vi "Measurement FileGLobal FGV.vi"(0 "New Measurements":T1, 2 "Enum":T2(ring), 11 "Error In":errorcluster) -> (4 "Combined Measurements":T1, 15 "Error Out":errorcluster)   [LabVIEW 2013]
uses:
  Controls/ks5080A_Measurements.ctl
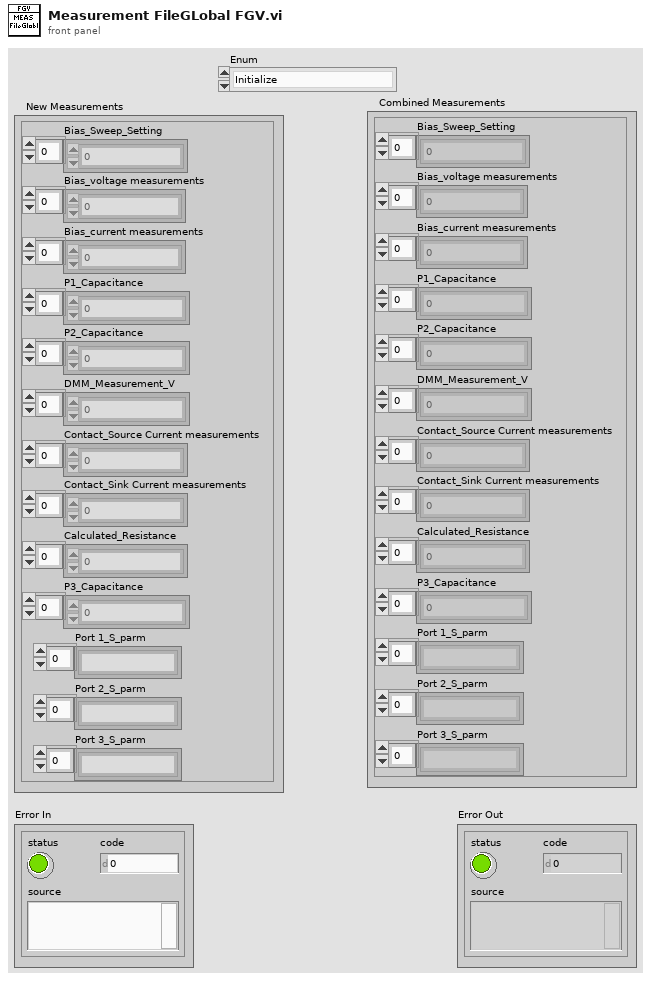
[diagram p1: front panel]
types:
  T1 = typedef "ks5080A_Measurements.ctl" = cluster{"Bias_Sweep_Setting":dbl[], "Bias_voltage measurements":dbl[], "Bias_current measurements":dbl[], "P1_Capacitance":dbl[], "P2_Capacitance":dbl[], "DMM_Measurement_V":dbl[], "Contact_Source Current measurements":dbl[], "Contact_Sink Current measurements":dbl[], "Calculated_Resistance":dbl[], "P3_Capacitance":dbl[], "Port 1_S_parm":string[], "Port 2_S_parm":string[], "Port 3_S_parm":string[]}
  T2 = enum16{"Initialize", "Insert Data into Array", "Get Data"}
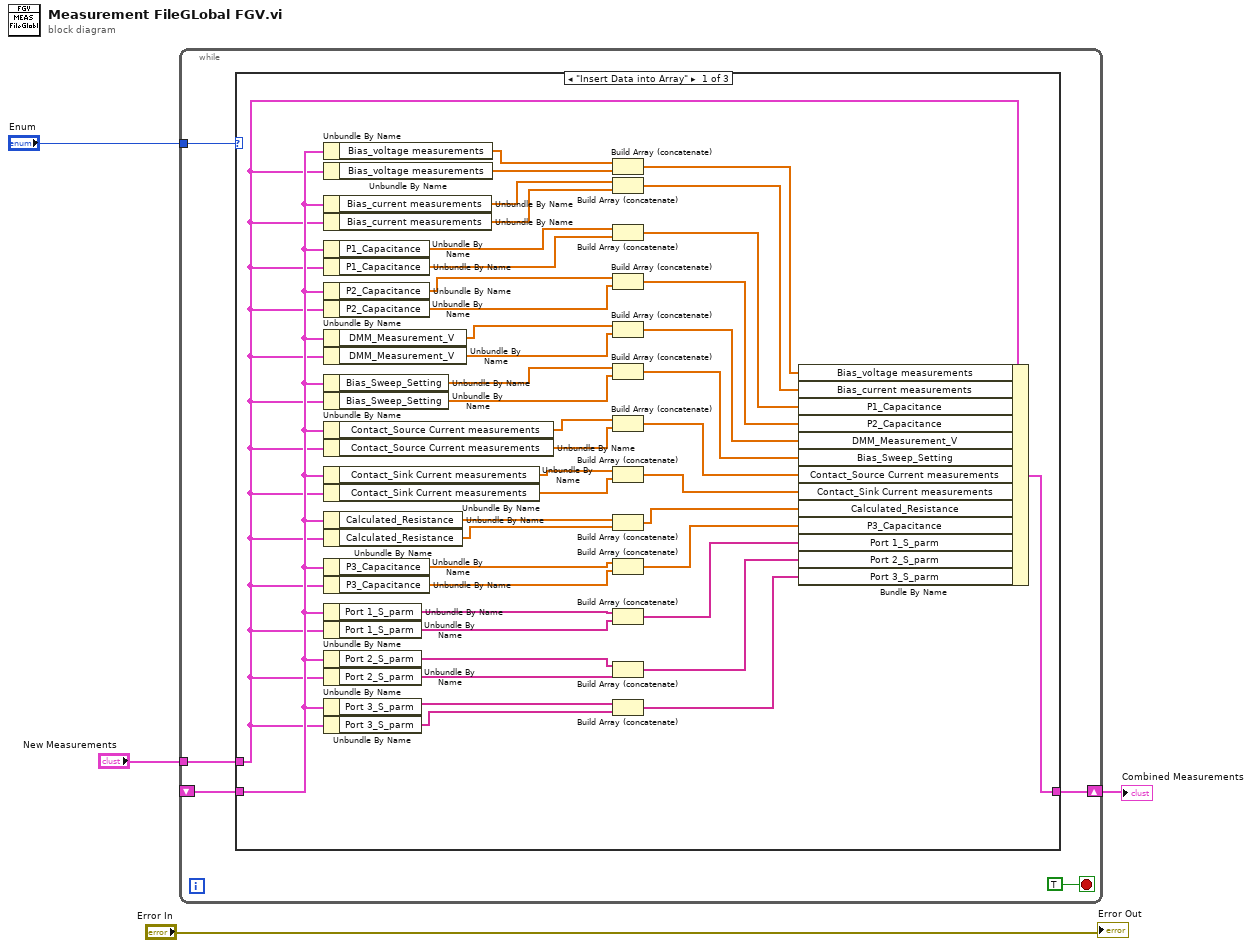
[diagram p0: block diagram]
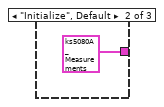
[diagram p2: hidden frame]
diagram:
  n1 = while {
    tunnel: "Enum" -> [w9]
    tunnel: "New Measurements" -> [w7]
    shift-right: [w6] -> w1
    shift-left: _ -> [w5]
    stop <- TRUE stop-if-true
    n2 = case shown="\"Insert Data into Array\"" w9 {
      tunnel: w7 -> [w10 _ _]
      tunnel: [w25 T1 {"Bias_Sweep_Setting"=[], "Bias_voltage measurements"=[], "Bias_current measurements"=[], "P1_Capacitance"=[], "P2_Capacitance"=[], "DMM_Measurement_V"=[], "Contact_Source Current measurements"=[], "Contact_Sink Current measurements"=[], "Calculated_Resistance"=[], "P3_Capacitance"=[], "Port 1_S_parm"=[], "Port 2_S_parm"=[], "Port 3_S_parm"=[]} ("ks5080A_Meaurements") w53] -> w6
      tunnel: w5 -> [w11 _ w53]
      frame "Insert Data into Array" {
        n3 = Unbundle By Name(w11) -> ("Bias_voltage measurements"=w51:dbl[])
        n4 = Unbundle By Name(w10) -> ("Bias_voltage measurements"=w50:dbl[])
        n5 = Unbundle By Name(w11) -> ("Bias_current measurements"=w48:dbl[])
        n6 = Unbundle By Name(w10) -> ("Bias_current measurements"=w47:dbl[])
        n7 = Unbundle By Name(w11) -> ("P1_Capacitance"=w45:dbl[])
        n8 = Unbundle By Name(w10) -> ("P1_Capacitance"=w43:dbl[])
        n9 = Unbundle By Name(w11) -> ("P2_Capacitance"=w42:dbl[])
        n10 = Unbundle By Name(w10) -> ("P2_Capacitance"=w41:dbl[])
        n11 = Unbundle By Name(w11) -> ("DMM_Measurement_V"=w38:dbl[])
        n12 = Unbundle By Name(w10) -> ("DMM_Measurement_V"=w37:dbl[])
        n13 = Unbundle By Name(w11) -> ("Bias_Sweep_Setting"=w35:dbl[])
        n14 = Unbundle By Name(w10) -> ("Bias_Sweep_Setting"=w36:dbl[])
        n15 = Unbundle By Name(w11) -> ("Contact_Source Current measurements"=w33:dbl[])
        n16 = Unbundle By Name(w10) -> ("Contact_Source Current measurements"=w32:dbl[])
        n17 = Unbundle By Name(w11) -> ("Contact_Sink Current measurements"=w30:dbl[])
        n18 = Unbundle By Name(w10) -> ("Contact_Sink Current measurements"=w29:dbl[])
        n19 = Unbundle By Name(w11) -> ("Calculated_Resistance"=w27:dbl[])
        n20 = Unbundle By Name(w10) -> ("Calculated_Resistance"=w26:dbl[])
        n21 = Unbundle By Name(w11) -> ("P3_Capacitance"=w24:dbl[])
        n22 = Unbundle By Name(w10) -> ("P3_Capacitance"=w23:dbl[])
        n23 = Unbundle By Name(w11) -> ("Port 1_S_parm"=w20:string[])
        n24 = Unbundle By Name(w10) -> ("Port 1_S_parm"=w19:string[])
        n25 = Unbundle By Name(w11) -> ("Port 2_S_parm"=w16:string[])
        n26 = Unbundle By Name(w10) -> ("Port 2_S_parm"=w15:string[])
        n27 = Unbundle By Name(w11) -> ("Port 3_S_parm"=w14:string[])
        n28 = Unbundle By Name(w10) -> ("Port 3_S_parm"=w13:string[])
        n29 = Build Array (concatenate)(w51, w50) -> (w49:dbl[])
        n30 = Build Array (concatenate)(w48, w47) -> (w46:dbl[])
        n31 = Build Array (concatenate)(w45, w43) -> (w44:dbl[])
        n32 = Build Array (concatenate)(w42, w41) -> (w40:dbl[])
        n33 = Build Array (concatenate)(w38, w37) -> (w39:dbl[])
        n34 = Build Array (concatenate)(w35, w36) -> (w34:dbl[])
        n35 = Build Array (concatenate)(w33, w32) -> (w31:dbl[])
        n36 = Build Array (concatenate)(w30, w29) -> (w28:dbl[])
        n37 = Build Array (concatenate)(w27, w26) -> (w22:dbl[])
        n38 = Build Array (concatenate)(w24, w23) -> (w21:dbl[])
        n39 = Build Array (concatenate)(w20, w19) -> (w18:string[])
        n40 = Build Array (concatenate)(w16, w15) -> (w17:string[])
        n41 = Build Array (concatenate)(w14, w13) -> (w12:string[])
        n42 = Bundle By Name(cluster=w10, "Bias_voltage measurements"=w49, "Bias_current measurements"=w46, "P1_Capacitance"=w44, "P2_Capacitance"=w40, "DMM_Measurement_V"=w39, "Bias_Sweep_Setting"=w34, "Contact_Source Current measurements"=w31, "Contact_Sink Current measurements"=w28, "Calculated_Resistance"=w22, "P3_Capacitance"=w21, "Port 1_S_parm"=w18, "Port 2_S_parm"=w17, "Port 3_S_parm"=w12) -> (w25:T1)
      }
      frame "Initialize", Default {
      }
      frame "Get Data" {
      }
    }
  }
  "Combined Measurements" <- w1
  "Error Out" <- "Error In"
